vi "GlobalSpeedUpdateTime.vi"() -> ()   [LabVIEW 2015]
panel:
  in  "Previous speed update time":dbl
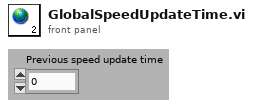
[diagram p1: front panel]
diagram:
